vi "IV_Sweep.vi"() -> ()   [LabVIEW 2016]
uses:
  <instrlib>/Keithley 24XX/Public/Data/Read (Single Point).vi
  <instrlib>/Keithley 24XX/Keithley 24XX.lvlib
panel:
  in  "Tab Control":enum32{"Voltage", "Current"}(tab)
  in  "Start (V)":dbl
  in  "End (V)":dbl=100.0
  in  "Compliance (A)":dbl=0.1
  in  "Interval (V)":dbl=100.0
  in  "Start (mA)":dbl
  in  "End (mA)":dbl=100.0
  in  "Compliance (V)":dbl=0.1
  in  "Interval (mA)":dbl=100.0
  in  "Output filename":path
  in  "2wire(F)/4wire(T)":bool
  out "IV":cluster{dbl[], dbl[]}(graph)
  out "Voltage":sgl=100.0186
  out "Current":sgl=-1.469503e-10
  out "Resistance":sgl=-680628800000.0
  in  "Delay Time (s)":dbl=1.0
  out "VR":cluster{dbl[], dbl[]}(graph)
  out "IR":cluster{dbl[], dbl[]}(graph)
  in  "Enable Resistance Auto Range (T:Enable)":bool=TRUE
  in  "Enable Current Auto Range (T:Enable)":bool=TRUE
  in  "Enable Voltage Auto Range (T:Enable)":bool=TRUE
  in  "Resistance Manual Range (1.0)":dbl=1.0
  in  "Current Manual Range (1.0)":dbl=1.0
  in  "Voltage Manual Range (1.0)":dbl=1.0
  in  "Serial Configuration":T1={"Baud Rate"=9600, "Parity"=0, "Data Bits"=8, "Stop Bits"=10, "Flow Control"=0} {"Flow Control" items=["None", "XON/XOFF", "RTS/CTS", "XON/XOFF & RTS/CTS", "DTR/DSR", "XON/XOFF & DTR/DSR"]; "Stop Bits" items=["1.0"=10, "1.5"=15, "2.0"=20]; "Data Bits" items=["7"=7, "8"=8]; "Parity" items=["None", "Odd", "Even", "Mark", "Space"]; "Baud Rate" items=["300"=300, "600"=600, "1200"=1200, "2400"=2400, "4800"=4800, "9600"=9600, "19200"=19200]}
  in  "VISA resource name":refnum<visa-resource-name>="COM5"
  # "Settings"
  # "I-V"
  # "V-R"
  # "I-R"
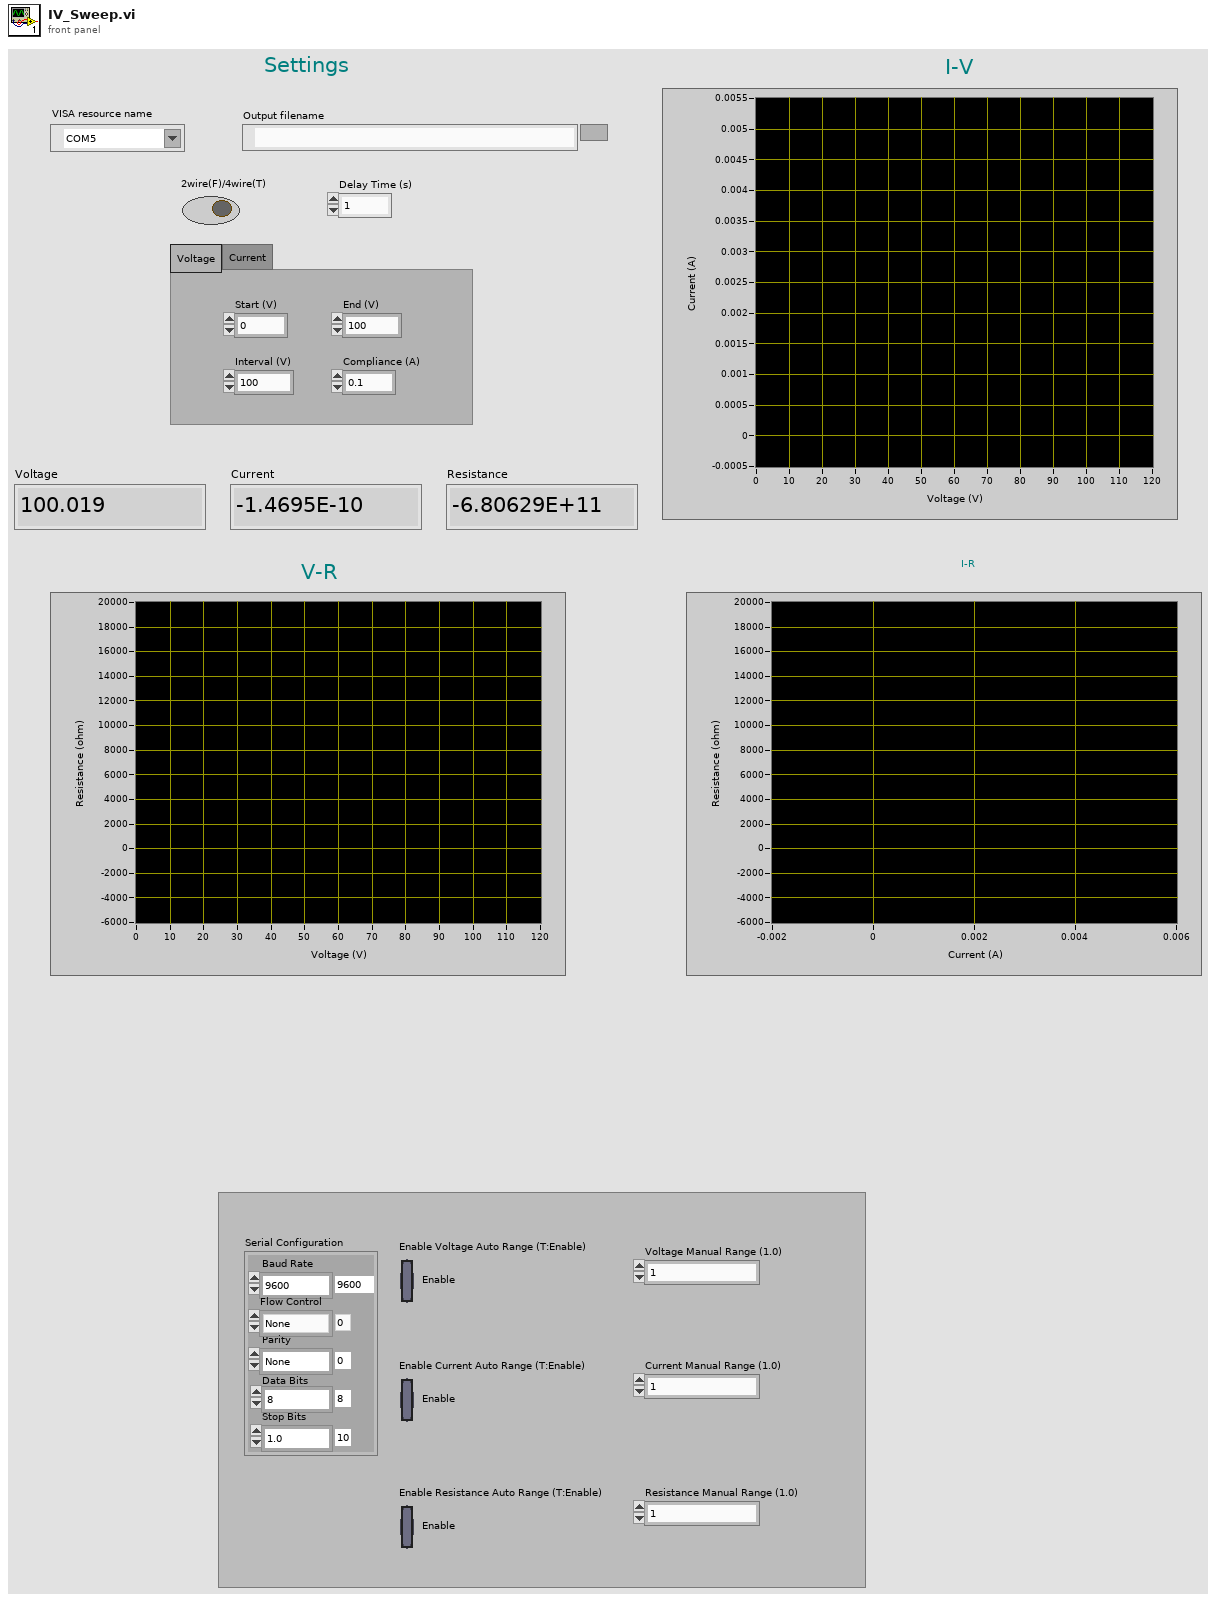
[diagram p1: front panel]
types:
  T1 = cluster{"Baud Rate":u32, "Parity":u16, "Data Bits":u16, "Stop Bits":u16, "Flow Control":u16}
  T2 = enum16{"open", "replace", "create", "open or create", "replace or create", "replace or create with confirmation"}
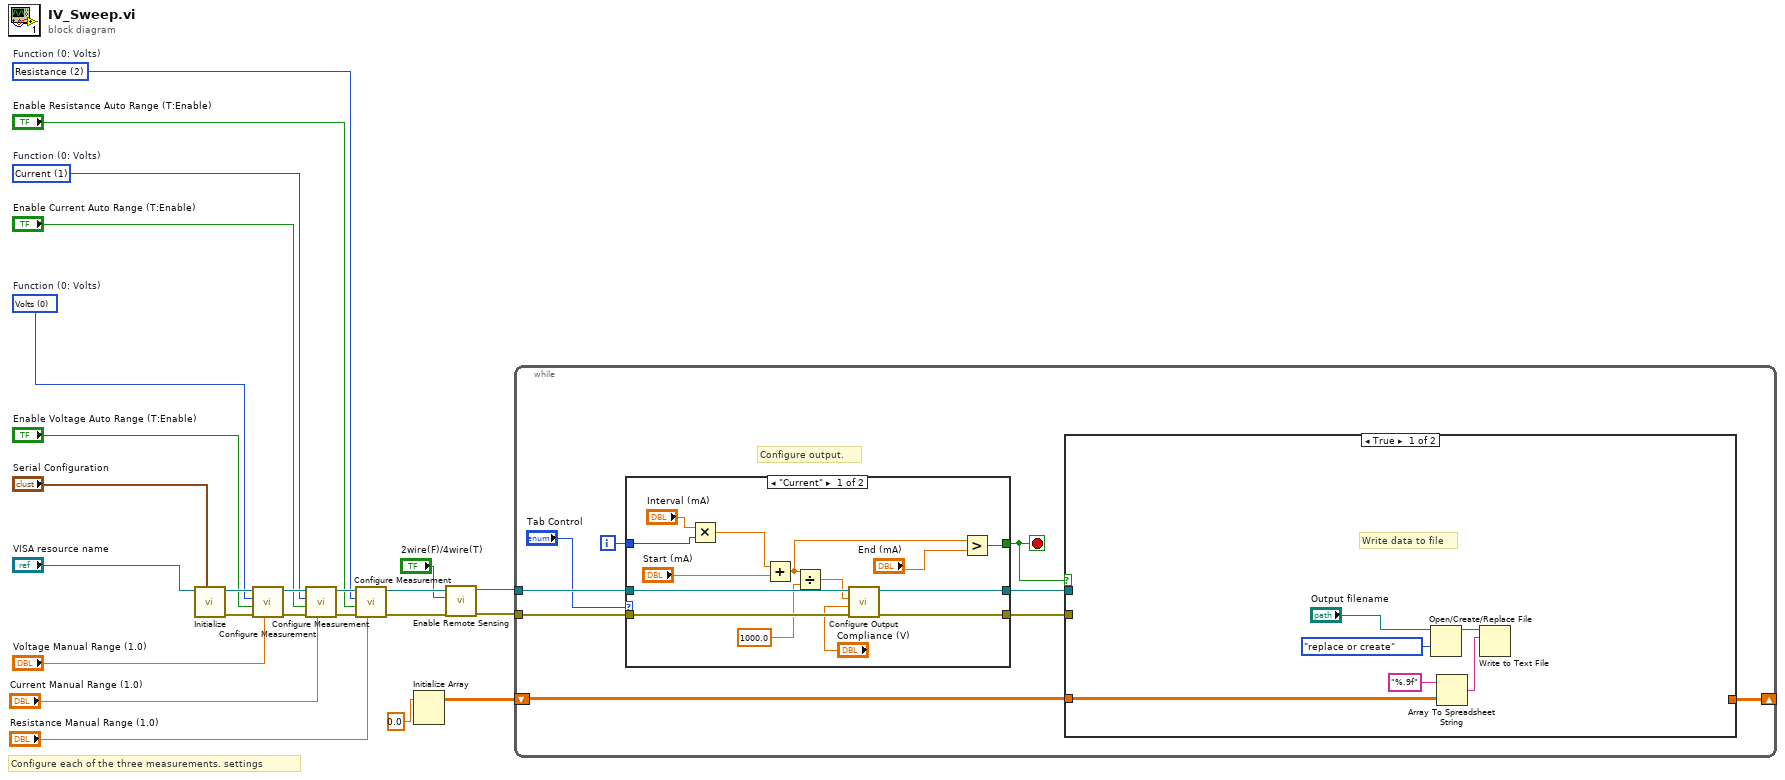
[diagram p0: block diagram]
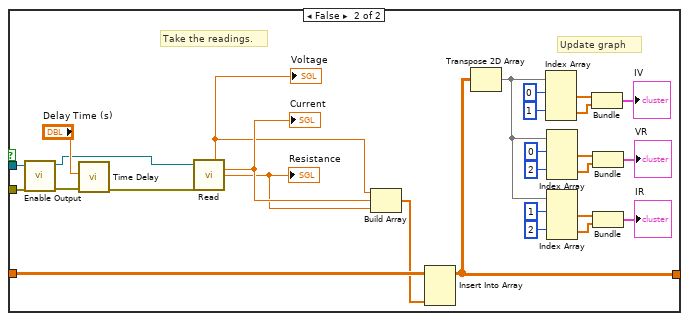
[diagram p2: hidden frame]
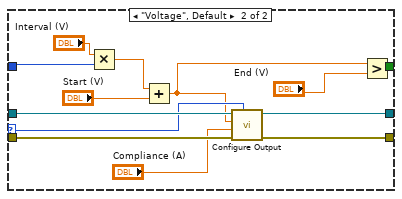
[diagram p3: hidden frame]
diagram:
  w14 = u16 2 items=["Volts", "Current", "Resistance"]  # Function (0: Volts)
  w15 = u16 1 items=["Volts", "Current", "Resistance"]  # Function (0: Volts)
  w16 = u16 0 items=["Volts", "Current", "Resistance"]  # Function (0: Volts)
  # "Configure each of the three measurements. settings"
  n1 = call <instrlib>:"Initialize.vi"("Serial Configuration"="Serial Configuration", "VISA resource name"="VISA resource name") -> ("error out"=w21:errorcluster, "VISA resource name out"=w22:refnum<visa-resource-name>)  [unwired: 8 in]
  n2 = call <instrlib>:"Configure Measurement.vi"("Manual Range (1.0)"="Voltage Manual Range (1.0)", "error in (no error)"=w21, "Enable Auto Range (T:Enable)"="Enable Voltage Auto Range (T:Enable)", "Function (0: Volts)"=w16, "VISA resource name"=w22) -> ("error out"=w19:errorcluster, "VISA resource name out"=w20:refnum<visa-resource-name>)  [unwired: 5 in]
  n3 = call <instrlib>:"Configure Measurement.vi"("Manual Range (1.0)"="Current Manual Range (1.0)", "error in (no error)"=w19, "Enable Auto Range (T:Enable)"="Enable Current Auto Range (T:Enable)", "Function (0: Volts)"=w15, "VISA resource name"=w20) -> ("error out"=w18:errorcluster, "VISA resource name out"=w17:refnum<visa-resource-name>)  [unwired: 5 in]
  n4 = call <instrlib>:"Configure Measurement.vi"("Manual Range (1.0)"="Resistance Manual Range (1.0)", "error in (no error)"=w18, "Enable Auto Range (T:Enable)"="Enable Resistance Auto Range (T:Enable)", "Function (0: Volts)"=w14, "VISA resource name"=w17) -> ("error out"=w4:errorcluster, "VISA resource name out"=w5:refnum<visa-resource-name>)  [unwired: 5 in]
  n5 = Initialize Array(0.0 ("element")) -> (w6:dbl[][])  [unwired: 2 in]
  n6 = call <instrlib>:"Enable Remote Sensing.vi"("error in (no error)"=w4, "Enable Remote Sensing (T: Enable)"="2wire(F)/4wire(T)", "VISA resource name"=w5) -> ("error out"=w2:errorcluster, "VISA resource name out"=w3:refnum<visa-resource-name>)  [unwired: 7 in]
  n7 = while {
    tunnel: w2 -> [w32]
    tunnel: w3 -> [w33]
    shift-right: [w30] -> _
    shift-left: w6 -> [w31]
    i -> [w26]
    stop <- w25 stop-if-true
    # "Configure output."
    n8 = case shown="\"Current\"" "Tab Control" {
      selector: "Tab Control" -> [_ w87]
      tunnel: w33 -> [w81 w94]
      tunnel: w32 -> [w80 w93]
      tunnel: [w78 w91] -> w29
      tunnel: [w77 w90] -> w28
      tunnel: [w73 w88] -> w25
      tunnel: w26 -> [w70 w84]
      frame "Current" {
        n9 = Multiply(x="Interval (mA)", y=w70) -> (x*y=w69:dbl)
        n10 = Add(x=w69, y="Start (mA)") -> (x+y=w72:dbl)
        n11 = Divide(x=w72, y=1000.0) -> (x/y=w74:dbl)
        n12 = call <instrlib>:"Configure Output.vi"("error in (no error)"=w80, "Compliance  Level (0.1)"="Compliance (V)", "Output Level (0)"=w74, "VISA resource name"=w81) -> ("error out"=w77:errorcluster, "VISA resource name out"=w78:refnum<visa-resource-name>)  [unwired: 6 in]
        n13 = Greater?(x=w72, y="End (mA)") -> (0:w73:bool)
      }
      frame "Voltage", Default {
        n14 = Multiply(x="Interval (V)", y=w84) -> (x*y=w83:dbl)
        n15 = Add(x=w83, y="Start (V)") -> (x+y=w82:dbl)
        n16 = call <instrlib>:"Configure Output.vi"("Source Mode  (0: Voltage)"=w87, "error in (no error)"=w93, "Compliance  Level (0.1)"="Compliance (A)", "Output Level (0)"=w82, "VISA resource name"=w94) -> ("error out"=w90:errorcluster, "VISA resource name out"=w91:refnum<visa-resource-name>)  [unwired: 5 in]
        n17 = Greater?(x=w82, y="End (V)") -> (0:w88:bool)
      }
    }
    n18 = case shown="True" w25 {
      tunnel: w31 -> [w34 w67]
      tunnel: [_ w63] -> w30
      tunnel: w29 -> [_ w56]
      tunnel: w28 -> [_ w54]
      frame True {
        # "Write data to file"
        n19 = Open/Create/Replace File(file path (use dialog)="Output filename", operation (0:open)=T2."replace or create") -> (refnum out=w38:refnum<file>)  [unwired: 4 in, 2 out]
        n20 = Array To Spreadsheet String(array=w34, 3:"%.9f" ("format string")) -> (spreadsheet string=w35:string)  [unwired: 1 in]
        n21 = Write to Text File(file (use dialog)=w38, text=w35) -> ()  [unwired: 2 in, 3 out]
      }
      frame False {
        # "Update graph"
        # "Take the readings."
        n22 = call <instrlib>:"Enable Output.vi"("error in (no error)"=w54, "VISA resource name"=w56) -> ("error out"=w53:errorcluster, "VISA resource name out"=w55:refnum<visa-resource-name>)  [unwired: 8 in]
        n23 = call "Time Delay"("error in (no error)"=w53, "Delay Time (s)"="Delay Time (s)") -> ("error out"=w59:errorcluster)  [unwired: 9 in]
        n24 = call-poly <instrlib>:"Read.vi"("VISA resource name"=w55, "error in (no error)"=w59) -> ("Voltage"=w60:sgl, "Current"=w61:sgl, "Resistance"=w57:sgl)  [unwired: 7 in, 4 out]
        "Voltage" <- w60
        "Current" <- w61
        "Resistance" <- w57
        n25 = Build Array(w60, w61, w57) -> (w62:sgl[])
        n26 = Insert Into Array(array=w67, new element=w62) -> (w63:dbl[][])  [unwired: 2 in]
        n27 = Transpose 2D Array(2D array=w63) -> (transposed array=w40:dbl[][])
        n28 = Index Array(array=w40, index (row) #1=0 ("index (row)"), index (row) #2=1 ("index (row)")) -> (element #1=w65:dbl[], element #2=w66:dbl[])  [unwired: 2 in]
        n29 = Index Array(array=w40, index (row) #1=0 ("index (row)"), index (row) #2=2 ("index (row)")) -> (element #1=w49:dbl[], element #2=w50:dbl[])  [unwired: 2 in]
        n30 = Index Array(array=w40, index (row) #1=1 ("index (row)"), index (row) #2=2 ("index (row)")) -> (element #1=w44:dbl[], element #2=w45:dbl[])  [unwired: 2 in]
        n31 = Bundle(w65, w66) -> (→"IV":cluster{dbl[], dbl[]})  [unwired: 1 in]
        n32 = Bundle(w49, w50) -> (→"VR":cluster{dbl[], dbl[]})  [unwired: 1 in]
        n33 = Bundle(w44, w45) -> (→"IR":cluster{dbl[], dbl[]})  [unwired: 1 in]
      }
    }
  }
